vi "Generic Read.vi"(8 "error in (no error)":errorcluster, 11 "Generic Instrument in":refnum<class "Generic Instrument.lvclass">) -> (0 "error out":errorcluster, 3 "Generic Instrument out":refnum<class "Generic Instrument.lvclass">)   [LabVIEW 2013]
uses:
  Generic Instrument.lvclass
panel:
  in  "VISA resource name":refnum<visa-resource-name>
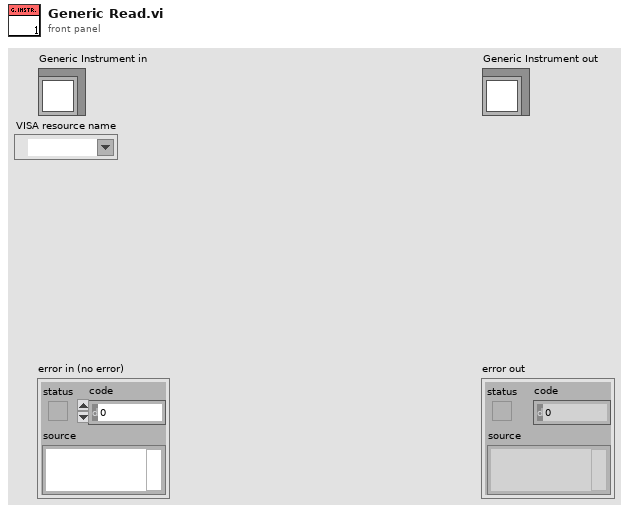
[diagram p1: front panel]
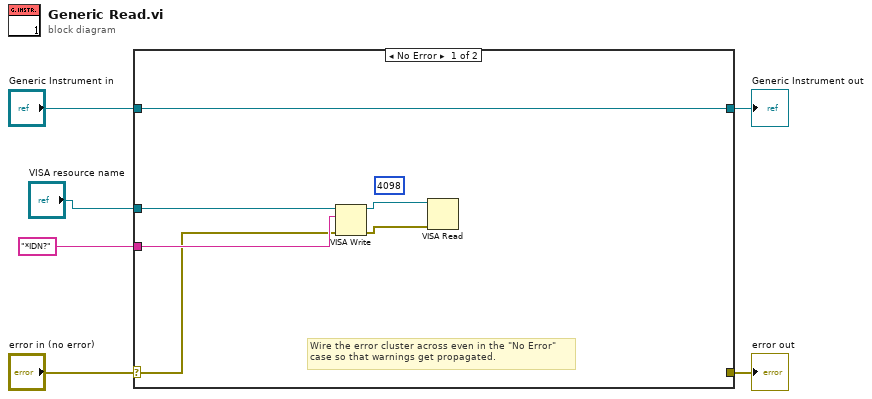
[diagram p0: block diagram]
diagram:
  n1 = case shown="No Error" "error in (no error)" {
    selector: "error in (no error)" -> [w9 w14]
    tunnel: [_ w14] -> w5
    tunnel: [w12 w13] -> w3
    tunnel: "Generic Instrument in" -> [w12 w13]
    tunnel: "VISA resource name" -> [w11 _]
    tunnel: "*IDN?" ("write buffer") -> [w10 _]
    frame No Error {
      (unwired) u32 4098 ("byte count")
      # "Wire the error cluster across even in the \"No Error\"\ncase so that warnings get propagated."
      n2 = VISA Write(VISA resource name=w11, write buffer=w10, error in (no error)=w9) -> (VISA resource name out=w8:refnum<visa-resource-name>, error out=w7:errorcluster)  [unwired: 1 out]
      n3 = VISA Read(VISA resource name=w8, error in (no error)=w7) -> ()  [unwired: 1 in, 4 out]
    }
    frame Error {
    }
  }
  "error out" <- w5
  "Generic Instrument out" <- w3
